vi "TestPcTcpSample.vi"() -> ()   [LabVIEW 2021]
doc: "ホール測定PC用TCP通信サンプル"
uses:
  SubVI/HallMeasurementStatus.ctl
  SubVI/TcpCommunicationClientCMD.ctl
panel:
  out "SettingFilePath":path
  out "TcpOK?":bool
  in  "Start":bool
  in  "DataFilePath":path=path "Test"
  out "SampleName":string
  in  "Status":T1
  out "ReadData":string
  in  "Send Data":string
  in  "Send":bool
  in  "ポート":u16=8501
  in  "中央PCアドレス":string="localhost"
  in  "停止":bool
  # "テストPC用TCP通信サンプル"
  # "1. マネージャーPC用TCP通信サンプル（ManagerTcpSample.exe）を実行します。\n\n2. テスト測定PC用TCP通信サンプル（TestTcpSample.exe）を実行します。\n　ManagerTcpSample.exeのリモートアドレスに、こちらのIPアドレスが表示されます。\n\n3. ManagerTcpSample.exeのエリプソ測定PCアドレスにアドレスを入力します。\n\n4. ManagerTcpSample.exeのボタンを押すと対応するコマンドが送られます。\n\n5. 受信したコマンドに応じて自動で返信を送信します。\n\n6. コマンドに対応してStatusやFilePath、StartやOKのLEDが変化します。\n\n7. 停止時はこちらのソフトを先に止めます。"
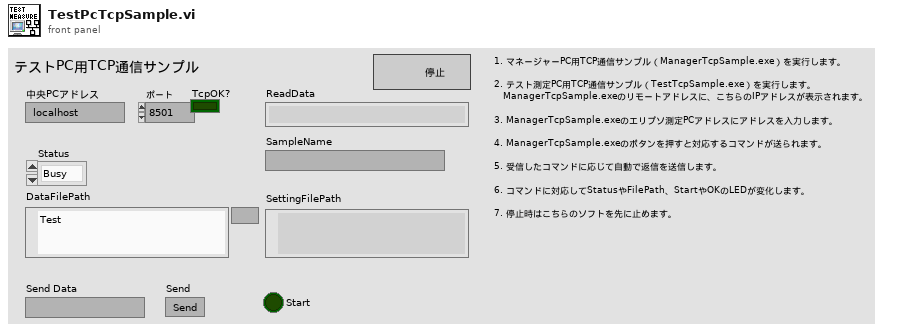
[diagram p1: front panel]
types:
  T1 = typedef "HallMeasurementStatus.ctl" = enum16{"Busy", "Ready", "Done", "Error"}
  T2 = typedef "TcpCommunicationClientCMD.ctl" = enum16{"Read", "Write", "Close"}
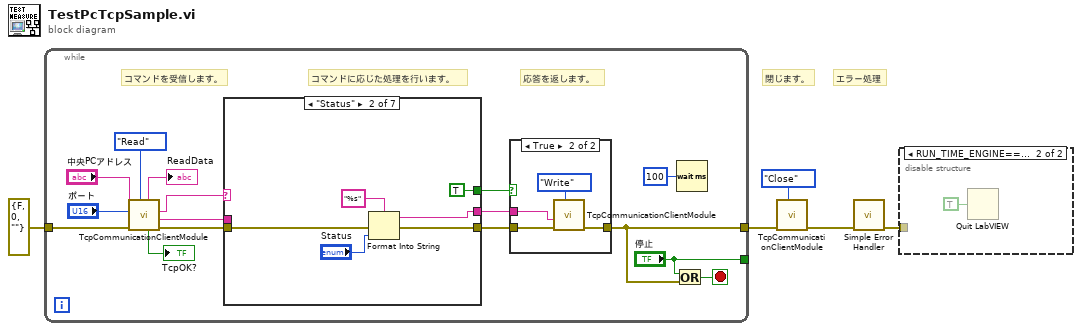
[diagram p0: block diagram]
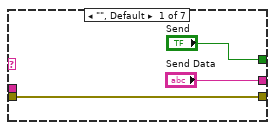
[diagram p4: hidden frame]
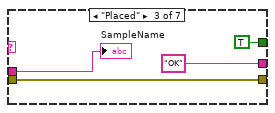
[diagram p5: hidden frame]
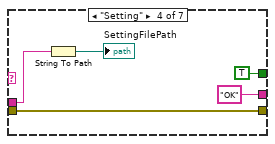
[diagram p6: hidden frame]
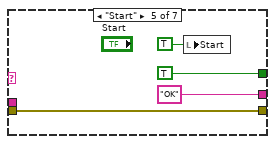
[diagram p7: hidden frame]
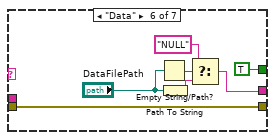
[diagram p8: hidden frame]
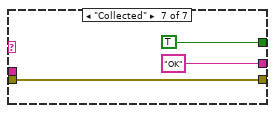
[diagram p9: hidden frame]
diagram:
  # "エラー処理"
  # "閉じます。"
  n1 = while {
    tunnel: ["停止"] -> _
    tunnel: [w10] -> w3
    tunnel: errorcluster {"status"=FALSE, "code"=0, "source"=""} ("エラー入力（エラーなし）") -> [w17]
    stop <- w21 stop-if-true
    # "応答を返します。"
    # "コマンドに応じた処理を行います。"
    # "コマンドを受信します。"
    n2 = call "TcpCommunicationClientModule.vi"("TcpCommunicationClientCMD"=TcpCommunicationClientCMD."Read", "エラー入力（エラーなし）"=w17, "ポート"="ポート", "アドレス"="中央PCアドレス") -> ("エラー出力"=w19:errorcluster, "Data"=w7:string, "Command"=w8:string, "TcpOK?"=→"TcpOK?":bool, "ReadData"=→"ReadData":string)  [unwired: 3 in]
    n3 = case shown="\"Status\"" w8 {
      tunnel: w7 -> [_ _ w36 w41 _ _ _]
      tunnel: ["Send Data" w34 "OK" ("Send Data") "OK" ("Send Data") "OK" ("Send Data") w50 "OK" ("Send Data")] -> w12
      tunnel: ["Send" TRUE ("Send") TRUE ("Send") TRUE ("Send") TRUE ("Send") TRUE ("Send") TRUE ("Send")] -> w13
      tunnel: w19 -> [w27 w32 w38 w42 w47 w54 w57]
      tunnel: [w27 w31 w38 w42 w47 w54 w57] -> w11
      frame "", Default {
      }
      frame "Status" {
        n4 = Format Into String(format string="%s" ("形式文字列"), error in=w32, "Status") -> (resulting string=w34:string, error out=w31:errorcluster)  [unwired: 1 in]
      }
      frame "Placed" {
        "SampleName" <- w36
      }
      frame "Setting" {
        n5 = String To Path(string=w41) -> (path=→"SettingFilePath":path)
      }
      frame "Start" {
        n6 = local write "Start"(TRUE) -> ()
      }
      frame "Data" {
        n7 = Empty String/Path?(string/path="DataFilePath") -> (empty?=w52:bool)
        n8 = Path To String(path="DataFilePath") -> (string=w51:string)
        n9 = Select(t="NULL", s=w52, f=w51) -> (s? t:f=w50:string)
      }
      frame "Collected" {
      }
    }
    n10 = case shown="True" w13 {
      tunnel: w11 -> [w22 w26]
      tunnel: [w22 w25] -> w10
      tunnel: w12 -> [_ w23]
      frame False {
      }
      frame True {
        n11 = call "TcpCommunicationClientModule.vi"("TcpCommunicationClientCMD"=TcpCommunicationClientCMD."Write", "エラー入力（エラーなし）"=w26, "WriteData"=w23) -> ("エラー出力"=w25:errorcluster)  [unwired: 4 in, 4 out]
      }
    }
    n12 = Or(x="停止", y=w10) -> (x .or. y?=w21:bool)
    n13 = Wait (ms)(milliseconds to wait=u32 100 ("ミリ秒待機時間")) -> ()  [unwired: 1 out]
  }
  n14 = call "TcpCommunicationClientModule.vi"("TcpCommunicationClientCMD"=TcpCommunicationClientCMD."Close", "エラー入力（エラーなし）"=w3) -> ("エラー出力"=w2:errorcluster)  [unwired: 5 in, 4 out]
  n15 = call <vilib>:"Simple Error Handler.vi"("error in (no error)"=w2) -> ("error out"=w1:errorcluster)  [unwired: 1 in, 7 out]
  n16 = disable-structure shown="RUN_TIME_ENGINE==True" {
    disable-tunnel: w1 -> [_ _]
    frame condition #0 (active) {
    }
    frame condition #1 {
      n17 = Quit LabVIEW(quit? (T)=TRUE) -> ()
    }
  }
